vi "Make Array Unique.vi"(11 "Array":string[](array[string])) -> (3 "Filtered Array":string[](array[string]))   [LabVIEW 2015, in "SLSC Switch.lvclass"]
uses:
  SLSC Switch.lvclass
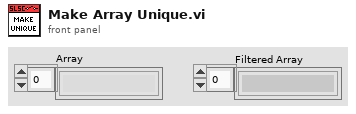
[diagram p1: front panel]
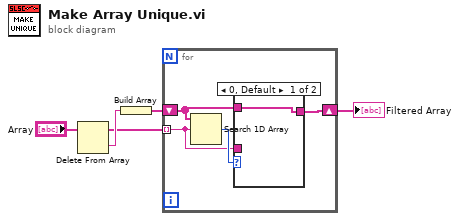
[diagram p0: block diagram]
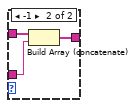
[diagram p2: hidden frame]
diagram:
  n1 = Delete From Array(array="Array") -> (deleted portion=w4:string, array with subset deleted=w3:string[])  [unwired: 2 in]
  n2 = Build Array(w4) -> (w1:string[])
  n3 = for {
    tunnel: w3 -> [w7] mode=indexing
    shift-right: [w6] -> w2
    shift-left: w1 -> [w8]
    n4 = Search 1D Array(1D array=w8, element=w7) -> (index of element=w9:i32)  [unwired: 1 in]
    n5 = case shown="0, Default" w9 {
      tunnel: w8 -> [w10 w13]
      tunnel: w7 -> [_ w12]
      tunnel: [w10 w11] -> w6
      frame 0, Default {
      }
      frame -1 {
        n6 = Build Array (concatenate)(w13, w12) -> (w11:string[])
      }
    }
  }
  "Filtered Array" <- w2
